vi "Handle Error Code.vi"(11 "Code":i32) -> (2 "error out":errorcluster)   [LabVIEW 2022 SP3, in "VoiceMeeterRemote.lvlib"]
uses:
  VoiceMeeterRemote.lvlib
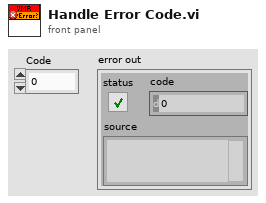
[diagram p1: front panel]
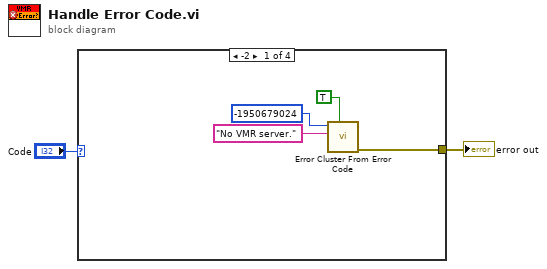
[diagram p0: block diagram]
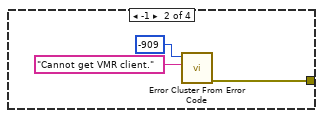
[diagram p2: hidden frame]
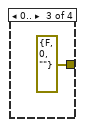
[diagram p3: hidden frame]
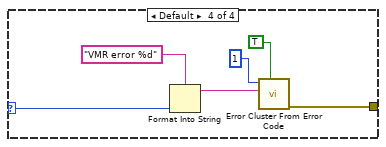
[diagram p4: hidden frame]
diagram:
  n1 = case shown="-2" "Code" {
    selector: "Code" -> [_ _ _ w14]
    tunnel: [w4 w7 errorcluster {"status"=FALSE, "code"=0, "source"=""} ("error out") w12] -> w1
    frame -2 {
      n2 = call <vilib>:"Error Cluster From Error Code.vi"("show call chain? (False)"=TRUE, "error message (\"\")"="No VMR server." ("error message (\"\")"), "error code (0)"=-1950679024) -> ("error out"=w4:errorcluster)  [unwired: 6 in]
    }
    frame -1 {
      n3 = call <vilib>:"Error Cluster From Error Code.vi"("error message (\"\")"="Cannot get VMR client." ("error message (\"\")"), "error code (0)"=-909) -> ("error out"=w7:errorcluster)  [unwired: 7 in]
    }
    frame 0.. {
    }
    frame Default {
      n4 = Format Into String(format string="VMR error %d", w14) -> (resulting string=w13:string)  [unwired: 2 in, 1 out]
      n5 = call <vilib>:"Error Cluster From Error Code.vi"("show call chain? (False)"=TRUE, "error message (\"\")"=w13, "error code (0)"=1) -> ("error out"=w12:errorcluster)  [unwired: 6 in]
    }
  }
  "error out" <- w1
